vi "Read and Update and Build.vi"(8 "error in (no error)":errorcluster, 11 "VIPM in":refnum<class "VIPM.lvclass">) -> (0 "error out":errorcluster, 3 "VIPM out":refnum<class "VIPM.lvclass">)   [LabVIEW 2019, in "VIPM.lvclass"]
uses:
  VIPM.lvclass
  VIPM.lvclass/VIPM.ctl
  <vilib>/JKI/VIPM API/VIPM API_vipm_api.lvlib
panel:
  out "Build Spec Summary":string="AH2500A 1.1.1.5\n\nProduct Description:\nLabVIEW drivers for Andeen-Hagerling 2500A capacitance bridge\n\nRelease Notes:\n[1.1.1]\n- Update to LV2019 and Instrument Framework v1.11.0\n\n---\n\nKrohn-Hite 7008 Drivers 1.7.3.33\n\nProduct Description:\nDrivers and control interface for Krohn-Hite 7008 multichannel amplifiers.\n\nRelease Notes:\n[1.7.3]\n- Update to Instrument Framework v1.11.0\n\n---\n\nLEIDEN TC 1.0.2.7\n\nProduct Description:\nTools used by LevyLab to interact with Leiden Temperature Control (TC)\n\n[Instrument.TC.MNK.lvclass]\n[Instrument.TC.CF.lvclass]\n- APIs that overrides \"Get Temperature.vi\" method of Instrument.Cryostat.lvclass\n\nRelease Notes:\n[1.0.2]\n- Fix CF Read T\n\n---\n\nCryostation 1.2.3.7\n\nProduct Description:\nProgram for logging Montana Instruments Cryostation status to the SQL DB. Provides a UI and API for getting information from the Cryostation.\n\nRelease Notes:\n[1.2.3]\n- Update to Instrument Framework v1.11.0\n\n---\n\nOxford-1820 1.3.3.23\n\nProduct Description:\nVIs for controlling the Oxford 18/20 magnet\n\nRelease Notes:\n- update to Instrument Framework v1.13.0\n\n---\n\nOxford-VRM 21.6.2.8\n\nProduct Description:\nVIs for controlling the Oxford VRM PS that controls the CF900's 3D magnet\n\nRelease Notes:\n[21.6.1]\n- Update to Instrument Framework v1.11.1\n\n---\n\nPPMS Monitor and Control 1.8.4.56\n\nProduct Description:\n- Log instrument status to the PGSQL database.\n- UI and API for controlling magnet field, temperature, and rotator angle (PPM2 only)\n\nRelease Notes:\n[1.8.4]\n- Update to Instrument Framework v1.11.1.15 (and SMO v1.4.0.69)\n- Fix Set methods\n\n---\n\nRazorbill RP100 21.2.3.9\n\nProduct Description:\nDivers for Razorbill RP100 HV amplifier\n\nRelease Notes:\n[21.2.4]\n- Update to  IF 1.11.1.15\n\n---\n"
  out "Path":path=path "C:/Users/patrick/Documents/GitHub/Razorbill-RP100/build support/Razorbill RP100.vipb"
  in  "Paths":path[](array[path])=[path "C:/Users/patrick/Documents/GitHub/Andeen-Hagerling-2500A/build support/AH2500A.vipb", path "C:/Users/patrick/Documents/GitHub/Krohn-Hite-7008/build support/Krohn Hite 7008.vipb", path "C:/Users/patrick/Documents/GitHub/Leiden-MNK-TC/build support/LEIDEN TC.vipb", path "C:/Users/patrick/Documents/GitHub/Montana-Instruments-Cryostation/build support/Cryostation.vipb", path "C:/Users/patrick/Documents/GitHub/Oxford-1820/build support/Oxford 1820 API.vipb", path "C:/Users/patrick/Documents/GitHub/Oxford-VRM/build support/Oxford VRM API.vipb", path "C:/Users/patrick/Documents/GitHub/PPMS-Monitor-and-Control/build support/PPMS Instrument.vipb", path "C:/Users/patrick/Documents/GitHub/Razorbill-RP100/build support/Razorbill RP100.vipb"]
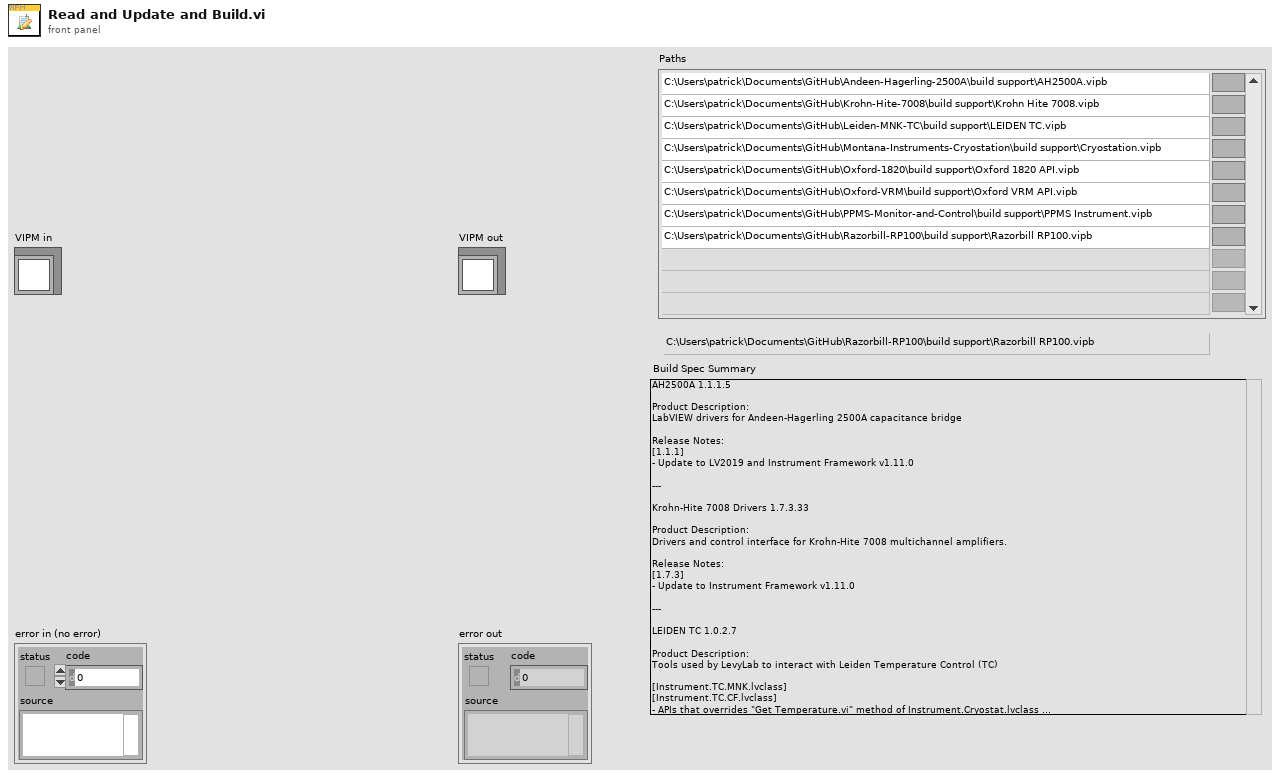
[diagram p1: front panel]
types:
  T1 = typedef "VIPM API_vipm_api.lvlib/VI Package Build Spec Data Cluster_vipm_api.ctl" = cluster{"Package Version":T2, "Product Name":string, "Company Name":string, "Author Name (Person or Company)":string, "Product Homepage (URL)":string, "Legal Copyright":string, "License Agreement Name":string, "Product Description Summary":string, "Product Description":string, "Release Notes - Change Log":string}
  T2 = typedef "VIPM API_vipm_api.lvlib/Version Info Cluster_vipm_api.ctl" = cluster{"major":u32, "minor":u32, "patch":u32, "build":u32}
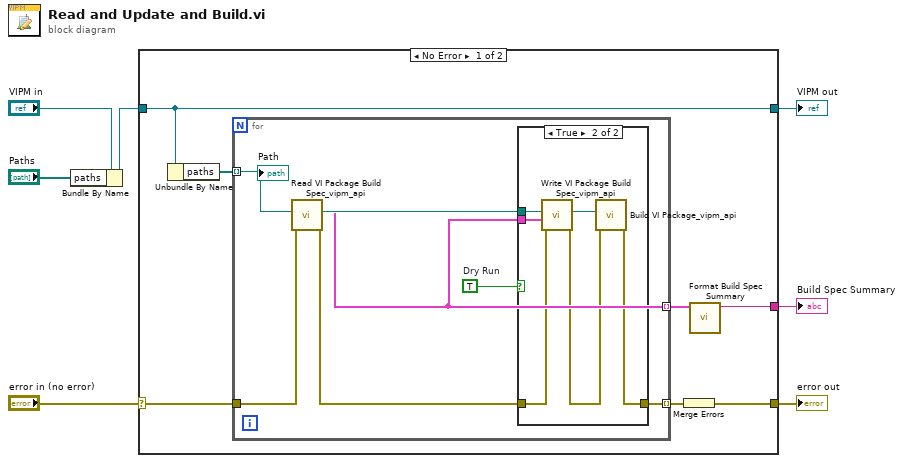
[diagram p0: block diagram]
diagram:
  n1 = Bundle By Name(cluster="VIPM in", "paths"="Paths") -> (w3:refnum<class "VIPM.lvclass">)
  n2 = case shown="No Error" "error in (no error)" {
    selector: "error in (no error)" -> [w12 w28]
    tunnel: [w10 w28] -> w6
    tunnel: [w14 w27] -> w5
    tunnel: w3 -> [w14 w27]
    tunnel: [w8 _] -> w1
    frame No Error {
      n3 = Unbundle By Name(w14) -> ("paths"=w13:path[])
      n4 = for {
        tunnel: w13 -> [w16] mode=indexing
        tunnel: w12 -> [w20]
        tunnel: [w18] -> w11 mode=indexing
        tunnel: [w15] -> w9 mode=indexing
        w17 = TRUE  # Dry Run
        n5 = call <vilib>:"Read VI Package Build Spec_vipm_api.vi"("error in (no error)"=w20, "Path to VIPB File"=w16) -> ("error out"=w19:errorcluster, "VI Package Build Spec Data"=w15:T1)  [unwired: 8 in]
        n6 = case shown="True" w17 {
          tunnel: w16 -> [_ w26]
          tunnel: w19 -> [w21 w25]
          tunnel: [w21 w24] -> w18
          tunnel: w15 -> [_ w22]
          frame False {
          }
          frame True {
            n7 = call <vilib>:"Write VI Package Build Spec_vipm_api.vi"("error in (no error)"=w25, "VI Package Build Spec Data"=w22, "Path to VIPB File"=w26) -> ("error out"=w23:errorcluster)  [unwired: 8 in]
            n8 = call <vilib>:"Build VI Package_vipm_api.vi"("error in (no error)"=w23, "Path to VIPB File"=w26) -> ("error out"=w24:errorcluster)  [unwired: 8 in, 1 out]
          }
        }
        "Path" <- w16
      }
      n9 = Merge Errors(w11) -> (w10:errorcluster)
      n10 = call "Format Build Spec Summary.vi"("Build Spec [] in"=w9) -> ("VIPB Preview"=w8:string)  [unwired: 10 in]
    }
    frame Error {
    }
  }
  "error out" <- w6
  "VIPM out" <- w5
  "Build Spec Summary" <- w1
